vi "HDF5 File Logging Example.vi"() -> ()   [LabVIEW 2014]
panel:
  in  "Dataset Path":string
  in  "Cooling Parameters":cluster{"dt":dbl, "T0":dbl, "Tf":dbl, "k":dbl}={"dt"=0.1, "T0"=10.0, "Tf"=1.0, "k"=0.1}
  in  "stop":bool
  out "Time Stamp":timestamp
  in  "File Path":path
  in  "Comment":string="Testing file writing"
  out "Waveform Chart":T1(graph)
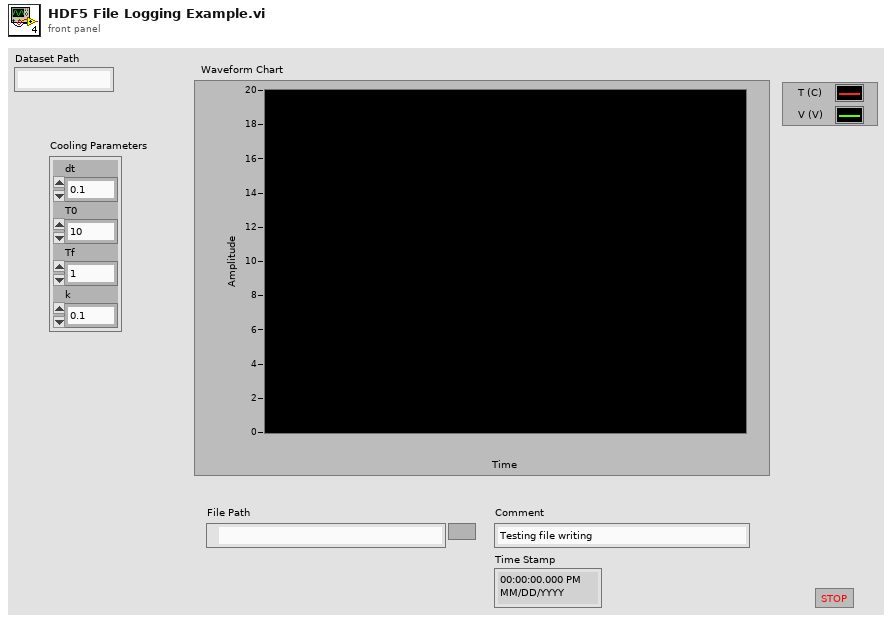
[diagram p1: front panel]
types:
  T1 = cluster{"Temperature (C)":dbl, "Voltage (V)":dbl}
  T2 = typedef "My Data HDF5 Refs.ctl" = cluster{"File Ref":T3, "Dataset Ref":T3}
  T3 = typedef "HDF5 Ref.ctl" = refnum<k1>
  T4 = cluster{"Time (s)":dbl, "Temperature (C)":dbl, "Voltage (V)":dbl}
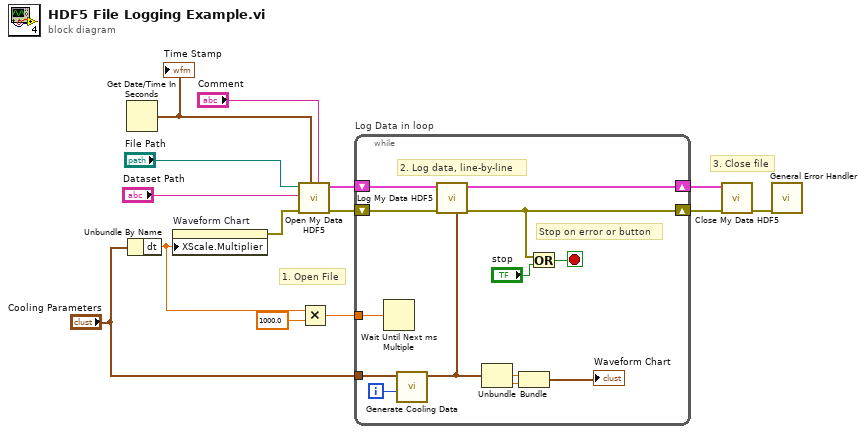
[diagram p0: block diagram]
diagram:
  # "3. Close file"
  # "1. Open File"
  n1 = Get Date/Time In Seconds() -> (seconds since 1Jan1904=w12:timestamp)
  "Time Stamp" <- w12
  n2 = Unbundle By Name("Cooling Parameters") -> ("dt"=w4:dbl)
  n3 = property on="Waveform Chart" class="WFChart (strict)"("XScale.Multiplier"=w4) -> (error out=w13:errorcluster)  [unwired: 2 in, 1 out]
  n4 = call "Open My Data HDF5.vi"("Comment"="Comment", "Time Stamp"=w12, "error in"=w13, "Dataset Path"="Dataset Path", "file path"="File Path") -> ("error out"=w9:errorcluster, "Refs"=w8:T2)  [unwired: 5 in]
  n5 = Multiply(x=w4, y=1000.0) -> (x*y=w2:dbl)
  n6 = while "Log Data in loop" {
    tunnel: "Cooling Parameters" -> [w26]
    shift-right: [w18] -> w7
    shift-left: w9 -> [w20]
    shift-right: [w17] -> w6
    shift-left: w8 -> [w15]
    tunnel: w2 -> [w16]
    i -> [w27]
    stop <- w21 stop-if-true
    # "2. Log data, line-by-line"
    # "Stop on error or button"
    n7 = Wait Until Next ms Multiple(millisecond multiple=w16) -> ()  [unwired: 1 out]
    n8 = call "Generate Cooling Data.vi"("i"=w27, "Cooling Parameters"=w26) -> ("Data"=w19:T4)  [unwired: 9 in]
    n9 = call "Log My Data HDF5.vi"("Data element"=w19, "error in"=w20, "Refs"=w15) -> ("error out"=w18:errorcluster, "Refs out"=w17:T2)  [unwired: 7 in]
    n10 = Unbundle(w19) -> ("Temperature (C)"=w25:dbl, "Voltage (V)"=w24:dbl)  [unwired: 1 out]
    n11 = Bundle("Temperature (C)"=w25, "Voltage (V)"=w24) -> (→"Waveform Chart":T1)  [unwired: 1 in]
    n12 = Or(x=w18, y="stop") -> (x .or. y?=w21:bool)
  }
  n13 = call "Close My Data HDF5.vi"("error in"=w7, "file refnum"=w6) -> ("error out"=w5:errorcluster)  [unwired: 9 in]
  n14 = call <vilib>:"General Error Handler.vi"("error in (no error)"=w5) -> ()  [unwired: 10 in, 5 out]
